vi "price.vi"(8 "error in (no error)":errorcluster, 11 "ColdDrink in":refnum<class "ColdDrink.lvclass">) -> (0 "error out":errorcluster, 2 "price":dbl, 3 "ColdDrink out":refnum<class "ColdDrink.lvclass">)   [LabVIEW 2017, in "ColdDrink.lvclass"]
uses:
  ColdDrink.lvclass
  Item Class/Item.lvclass
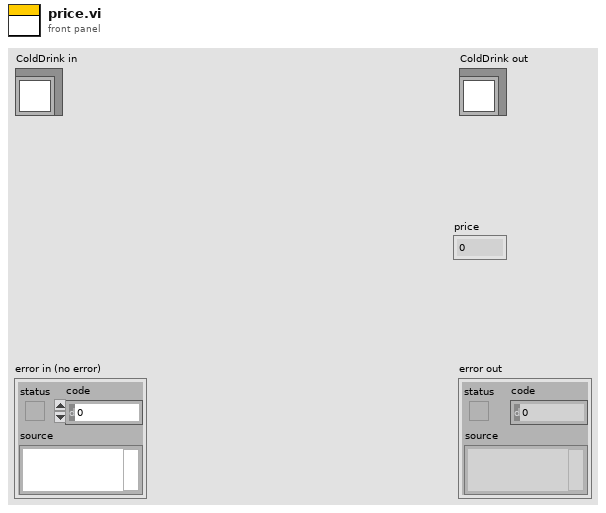
[diagram p1: front panel]
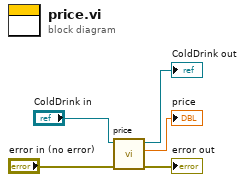
[diagram p0: block diagram]
diagram:
  n1 = call-parent "price.vi"("error in (no error)"="error in (no error)", "Item in"="ColdDrink in") -> ("error out"=→"error out":errorcluster, "price"=→"price":dbl, "Item out"=→"ColdDrink out":refnum<class "ColdDrink.lvclass">)  [unwired: 7 in]
